vi "Mutate Settings and Memory Channel.vi"(8 "error in (no error)":errorcluster, 11 "Item Ref in":T1 format="%.0x") -> (0 "error out":errorcluster, 3 "Item Ref out":T1 format="%.0x")   [LabVIEW 2027, in "System Monitor System Explorer.lvlib"]
uses:
  System Monitor System Explorer.lvlib
  <vilib>/NI VeriStand/Custom Device API/Custom Device Item Ref.ctl
  Shared/System Monitor Settings.ctl
  <vilib>/NI VeriStand/Custom Device API/Get Item Property (Variant).vi
  <vilib>/NI VeriStand/Custom Device API/Custom Device API.lvlib
  Shared/System Monitor Shared.lvlib
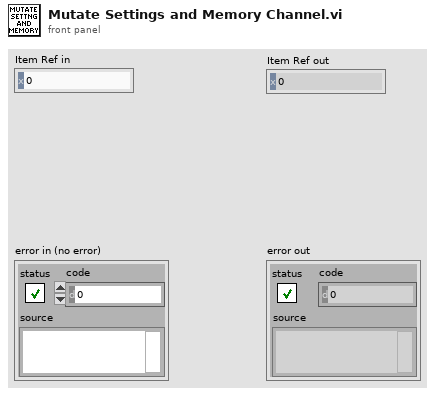
[diagram p1: front panel]
types:
  T1 = typedef "Custom Device API.lvlib/Custom Device Item Ref.ctl" = u64
  T2 = typedef "System Monitor Shared.lvlib/System Monitor Settings.ctl" = cluster{"Number of CPU Cores":u64, "Update Rate (Hz)":dbl}
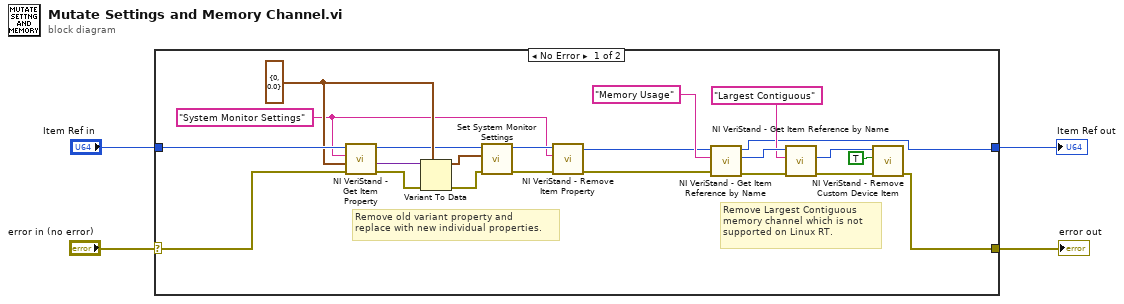
[diagram p0: block diagram]
diagram:
  n1 = case shown="No Error" "error in (no error)" {
    selector: "error in (no error)" -> [w25 w27]
    tunnel: [w10 w27] -> w3
    tunnel: [w11 w28] -> w2
    tunnel: "Item Ref in" -> [w26 w28]
    frame No Error {
      w22 = T2 {"Number of CPU Cores"=0, "Update Rate (Hz)"=0.0} ("System Monitor Settings")
      w7 = "System Monitor Settings" ("Property Name")
      # "Remove Largest Contiguous\nmemory channel which is not\nsupported on Linux RT."
      # "Remove old variant property and\nreplace with new individual properties."
      n2 = call-poly <vilib>:"NI VeriStand - Get Item Property.vi"("error in (no error)"=w25, "Default Value"=w22, "Property Name"=w7, "Item Ref in"=w26) -> ("error out"=w24:errorcluster, "Value"=w23:variant, "Item Ref out"=w19:T1)  [unwired: 4 in, 1 out]
      n3 = Variant To Data(error in=w24, type=w22, Variant=w23) -> (data=w21:T2, error out=w20:errorcluster)
      n4 = call "Set System Monitor Settings.vi"("error in (no error)"=w20, "System Monitor Settings"=w21, "Item Ref in"=w19) -> ("error out"=w9:errorcluster, "Item Ref out"=w8:T1)  [unwired: 7 in]
      n5 = call <vilib>:"NI VeriStand - Remove Item Property.vi"("error in (no error)"=w9, "Property Name"=w7, "Item Ref in"=w8) -> ("error out"=w6:errorcluster, "Item Ref out"=w5:T1)  [unwired: 6 in, 1 out]
      n6 = call <vilib>:"NI VeriStand - Get Item Reference by Name.vi"("error in (no error)"=w6, "Item Name"="Memory Usage" ("Section Name"), "Parent Ref in"=w5) -> ("error out"=w15:errorcluster, "Item Ref"=w17:T1, "Parent Ref out"=w11:T1)  [unwired: 5 in, 1 out]
      n7 = call <vilib>:"NI VeriStand - Get Item Reference by Name.vi"("error in (no error)"=w15, "Item Name"="Largest Contiguous" ("Section Name"), "Parent Ref in"=w17) -> ("error out"=w12:errorcluster, "Item Ref"=w14:T1)  [unwired: 5 in, 2 out]
      n8 = call <vilib>:"NI VeriStand - Remove Custom Device Item.vi"("error in (no error)"=w12, "Force Delete (F)"=TRUE, "Item Ref in"=w14) -> ("error out"=w10:errorcluster)  [unwired: 7 in, 1 out]
    }
    frame Error {
    }
  }
  "error out" <- w3
  "Item Ref out" <- w2
